vi "He magnet field fpga.vi"() -> ()   [LabVIEW 2016]
uses:
  <vilib>/LabVIEW Targets/FPGA/cRIO/shared/nicrio_ModuleControls/nicrio_cRIO-9871_BaudRateEnum.ctl
  <vilib>/LabVIEW Targets/FPGA/cRIO/shared/nicrio_ModuleControls/nicrio_cRIO-9871_DataBitsEnum.ctl
  <vilib>/LabVIEW Targets/FPGA/cRIO/shared/nicrio_ModuleControls/nicrio_cRIO-9871_ParityEnum.ctl
  <vilib>/LabVIEW Targets/FPGA/cRIO/shared/nicrio_ModuleControls/nicrio_cRIO-9871_StopBitsEnum.ctl
  <vilib>/Platform/TimedLoop/XDataNode/timing_clust.ctl
  <vilib>/Platform/TimedLoop/XDataNode/nitl_modes.ctl
  <vilib>/Platform/TimedLoop/XDataNode/wakeup.ctl
  <vilib>/rvi/FXPMathLib/basic elements/FxpIntAccumulator/subVIs/nifxpmath_IntAccumulator_SimConfig.ctl
  <vilib>/rvi/Emulation/niFpgaGetClockAttributes.vi
  <vilib>/rvi/Emulation/niFpgaSctlEmulationGetInTimedLoop.vi
  <vilib>/rvi/Emulation/niFpgaEmulationReportErrorSimple.vi
  <vilib>/rvi/eio/common/nirviEmuTemplateMethod_errors.vi
  <vilib>/rvi/Emulation/niFpgaCriticalErrorInLSC.vi
  <vilib>/rvi/Analysis/common/codeGenErrors/XNode/niFpgaXNodeCodeGenErrorHandle.vi
  <vilib>/rvi/FXPMathLib/basic elements/FxpIntAccumulator/simVIs/DllFxpIntAccumulator_sub.vi
  <vilib>/rvi/eio/common/nirviEmuTemplatePropertySet_noerrors.vi
  <vilib>/eio/EIONode/EIONode.xnode
  <vilib>/eio/EIOMethodNode/EIOMethodNode.xnode
  <vilib>/rvi/Analysis/measure/dc-rms/XNode/niFpgaDC-RMS.xnode
  <vilib>/Platform/TimedLoop/XDataNode/XDataNode.xnode
  <vilib>/rvi/FXPMathLib/basic elements/FxpIntAccumulator/XNode/nifxpmath_IntAccumulator.xnode
  <vilib>/rvi/FXPMathLib/FxpMul/XNode/nifxpmath_Multiplier.xnode
  <vilib>/eio/EIOPropertyNode/EIOPropertyNode.xnode
  <vilib>/Platform/TimedLoop/XDataNode/XDNodeRunTimeDep.lvlib
  <vilib>/rvi/FXPMathLib/sim/FxpSim.dll
  <vilib>/rvi/eio/common/nirviEmuTemplatePropertyGet_errors.vi
  <vilib>/rvi/eio/common/nirviEmuTemplatePropertyGet_noerrors.vi
  <vilib>/rvi/eio/common/nirviEmuTemplatePropertySet_errors.vi
panel:
  out "Ion gauge 4":u8[](array[numeric])
  out "Convectron 4":u8[](array[numeric])
  out "Convectron 3":u8[](array[numeric])
  out "Ion gauge 3":u8[](array[numeric])
  out "Ion gauge 2":u8[](array[numeric])
  out "Convectron 2":u8[](array[numeric])
  out "Convectron 1":u8[](array[numeric])
  out "Ion gauge 1":u8[](array[numeric])
  in  "Analyze Image FC":bool
  in  "Tank Exit FC":bool
  out "Analyze Out?":bool
  out "Analyze IN?":bool
  in  "Analog Output":fxp<+/-,26,5>[](array[numeric])=[0.0, 0.0, 0.0, 0.0, 0.0, 0.0, 0.0, 0.0] format="%.23g"
  out "Analog input":fxp<+/-,26,5>[](array[numeric]) format="%.23g"
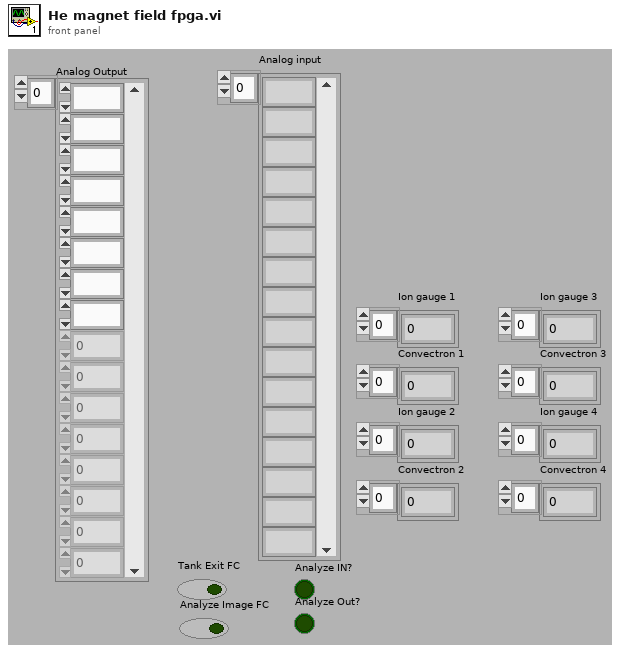
[diagram p1: front panel]
types:
  T1 = typedef "nicrio_cRIO-9871_StopBitsEnum.ctl" = enum8{"1", "1.5", "2"}
  T2 = typedef "nicrio_cRIO-9871_ParityEnum.ctl" = enum8{"None", "Odd", "Even", "Mark", "Space"}
  T3 = typedef "nicrio_cRIO-9871_DataBitsEnum.ctl" = enum8{"5", "6", "7", "8"}
  T4 = typedef "nicrio_cRIO-9871_BaudRateEnum.ctl" = enum16{"75 bps", "110 bps", "134 bps", "150 bps", "300 bps", "600 bps", "1200 bps", "1800 bps", "2400 bps", "4800 bps", "7200 bps", "9600 bps", "14.4 kbps", "19.2 kbps", "28.8 kbps", "38.4 kbps", "57.6 kbps", "115.2 kbps", "230.4 kbps", "460.8 kbps", "921.6 kbps"}
  T5 = typedef "XDNodeRunTimeDep.lvlib/timing_clust.ctl" = cluster{"Expected End [f-1]":u64, "Actual End [f-1]":u64, "Finished Late? [f-1]":bool, "Expected End [i-1]":u64, "Actual End [i-1]":u64, "Finished Late? [i-1]":bool, "Expected Start [i]":u64, "Actual Start [i]":u64, "Expected Start [f]":u64, "Actual Start [f]":u64, "Source Name":string, "Structure Name":string, "Period":i64, "Deadline":i64, "Offset":i64, "Start":i64, "Priority":i32, "Timeout":i32, "Mode":T6, "Wakeup Reason":T7, "Error":errorcluster, "Source Type":string, "Secondary Source Type":string, "Global End Time":u64, "Global Start Time":u64, "Frame Duration":u64, "Iteration Duration":u64, "Assigned CPU":i32, "I/O Scan Engine Mode":u32}
  T6 = typedef "XDNodeRunTimeDep.lvlib/nitl_modes.ctl" = enum32{"No Change", "Process missed periods, maintain original phase", "Discard missed periods, maintain original phase", "Process missed periods, ignore original phase", "Discard missed periods, ignore original phase"}
  T7 = typedef "XDNodeRunTimeDep.lvlib/wakeup.ctl" = enum32{"Normal", "Aborted", "Asynchronous wakeup", "Timing source error", "Timed loop error", "Timeout"}
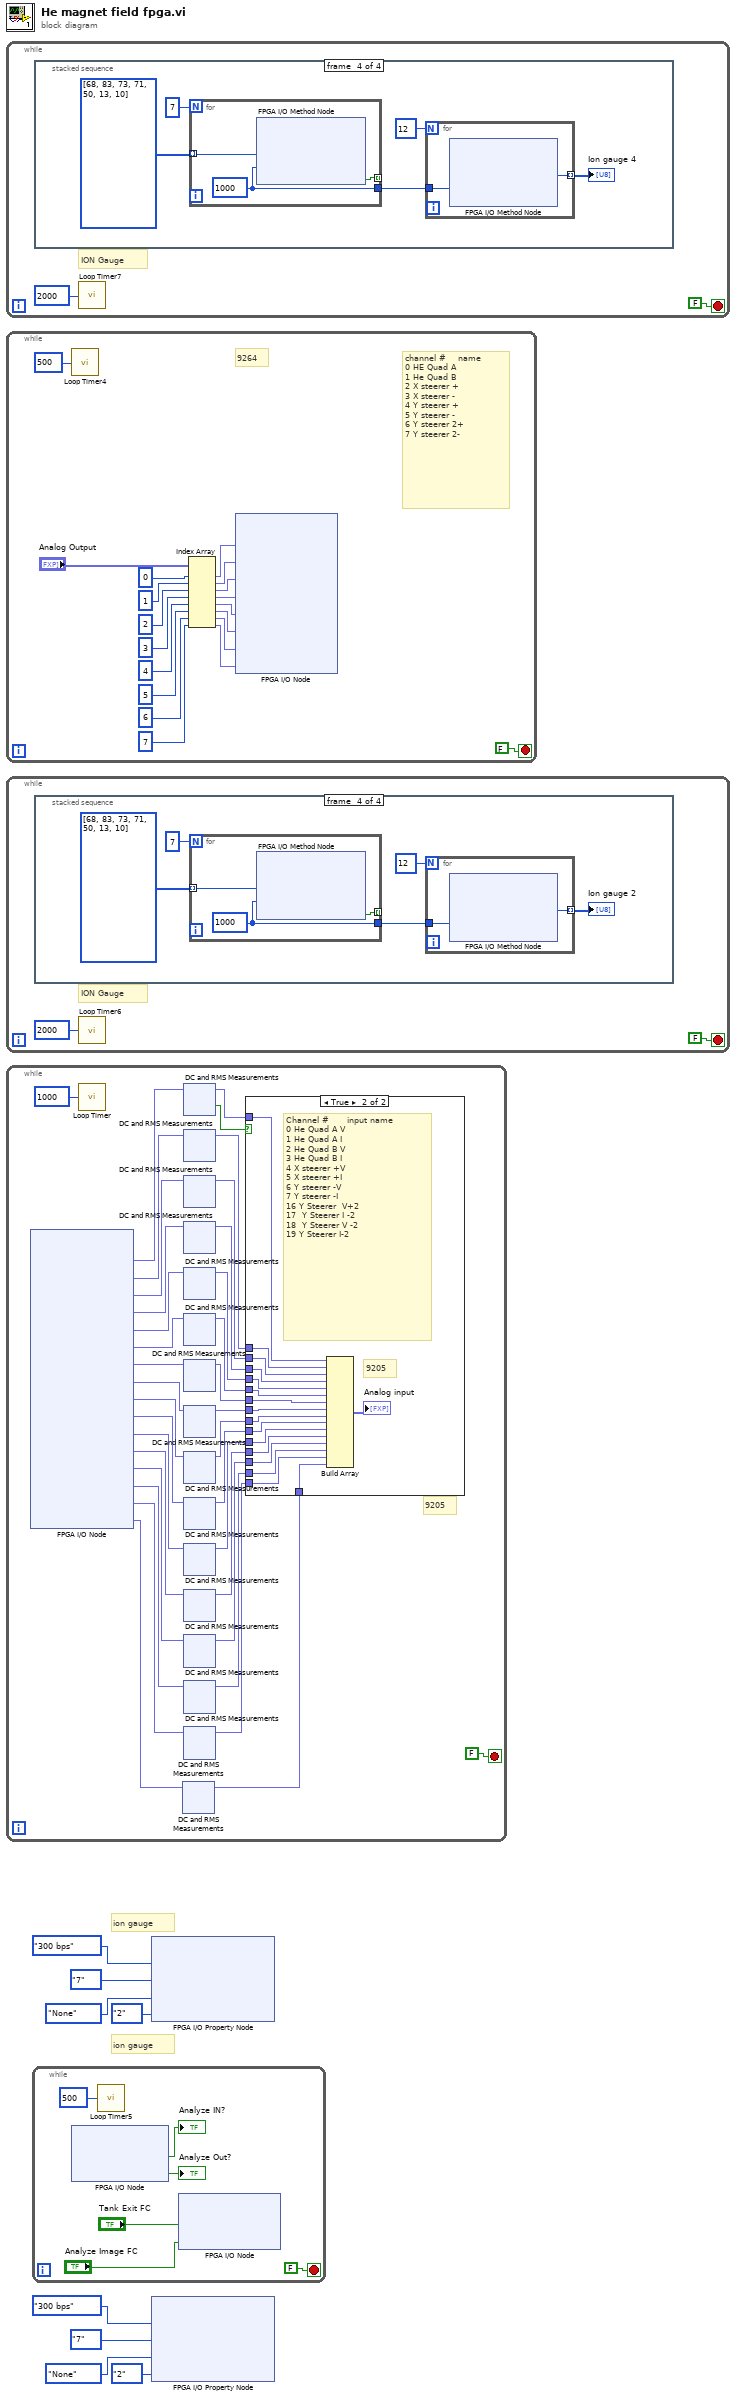
[diagram p0: block diagram]
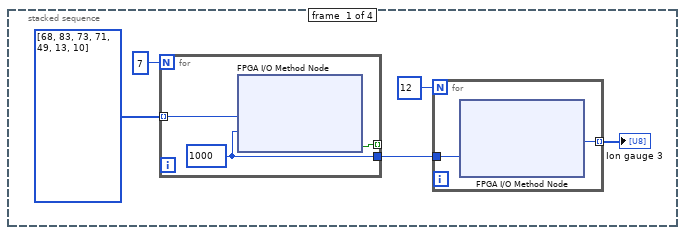
[diagram p3: hidden frame]
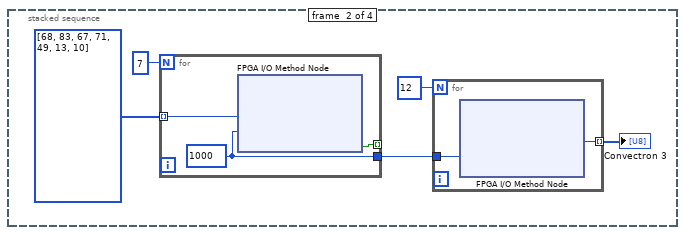
[diagram p4: hidden frame]
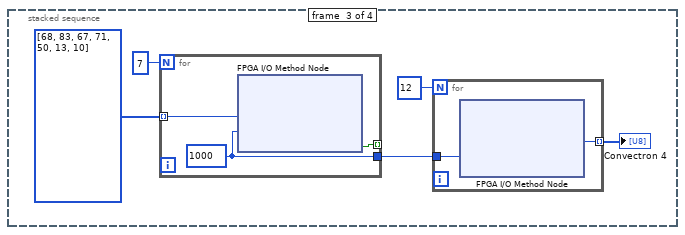
[diagram p5: hidden frame]
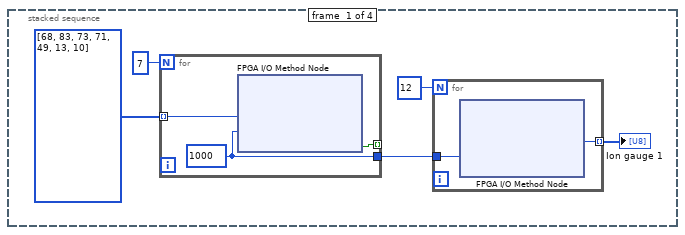
[diagram p6: hidden frame]
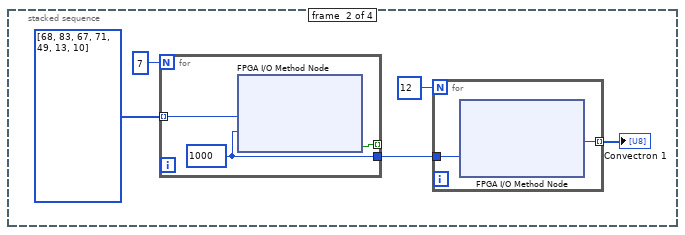
[diagram p7: hidden frame]
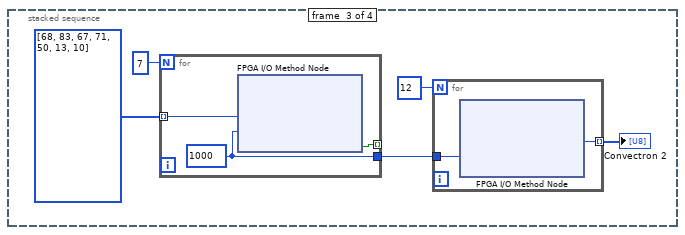
[diagram p8: hidden frame]
diagram:
  # "ion gauge"
  # "ion gauge"
  n1 = while {
    stop <- FALSE stop-if-true
    # "ION Gauge"
    n2 = stacked-sequence {
      frame #0 {
        n3 = for {
          N: 7 -> [_]
          tunnel: [w18] -> w15
          tunnel: [w19] -> _ mode=indexing
          tunnel: u8[] [68, 83, 73, 71, 49, 13, 10] ("unsigned byte array") -> [w20] mode=indexing
          w18 = 1000 ("Timeout (ms)")
          n4 = xnode "FPGA I/O Method Node"("Data"=w20, "Timeout (ms)"=w18) -> ("Timed Out"=w19:bool)  [unwired: 1 in, 1 out]
        }
        n5 = for {
          N: 12 -> [_]
          tunnel: w15 -> [w17]
          tunnel: [w16] -> w11 mode=indexing
          n6 = xnode "FPGA I/O Method Node"("Timeout (ms)"=w17) -> ("Data"=w16:u8)  [unwired: 1 in, 2 out]
        }
        "Ion gauge 3" <- w11
      }
      frame #1 {
        n7 = for {
          N: 7 -> [_]
          tunnel: [w29] -> w25
          tunnel: [w28] -> _ mode=indexing
          tunnel: u8[] [68, 83, 67, 71, 49, 13, 10] ("unsigned byte array") -> [w30] mode=indexing
          w29 = 1000 ("Timeout (ms)")
          n8 = xnode "FPGA I/O Method Node"("Data"=w30, "Timeout (ms)"=w29) -> ("Timed Out"=w28:bool)  [unwired: 1 in, 1 out]
        }
        n9 = for {
          N: 12 -> [_]
          tunnel: w25 -> [w26]
          tunnel: [w27] -> w21 mode=indexing
          n10 = xnode "FPGA I/O Method Node"("Timeout (ms)"=w26) -> ("Data"=w27:u8)  [unwired: 1 in, 2 out]
        }
        "Convectron 3" <- w21
      }
      frame #2 {
        n11 = for {
          N: 7 -> [_]
          tunnel: [w38] -> w35
          tunnel: [w39] -> _ mode=indexing
          tunnel: u8[] [68, 83, 67, 71, 50, 13, 10] ("unsigned byte array") -> [w40] mode=indexing
          w38 = 1000 ("Timeout (ms)")
          n12 = xnode "FPGA I/O Method Node"("Data"=w40, "Timeout (ms)"=w38) -> ("Timed Out"=w39:bool)  [unwired: 1 in, 1 out]
        }
        n13 = for {
          N: 12 -> [_]
          tunnel: w35 -> [w37]
          tunnel: [w36] -> w31 mode=indexing
          n14 = xnode "FPGA I/O Method Node"("Timeout (ms)"=w37) -> ("Data"=w36:u8)  [unwired: 1 in, 2 out]
        }
        "Convectron 4" <- w31
      }
      frame #3 {
        n15 = for {
          N: 7 -> [_]
          tunnel: [w49] -> w45
          tunnel: [w48] -> _ mode=indexing
          tunnel: u8[] [68, 83, 73, 71, 50, 13, 10] ("unsigned byte array") -> [w50] mode=indexing
          w49 = 1000 ("Timeout (ms)")
          n16 = xnode "FPGA I/O Method Node"("Data"=w50, "Timeout (ms)"=w49) -> ("Timed Out"=w48:bool)  [unwired: 1 in, 1 out]
        }
        n17 = for {
          N: 12 -> [_]
          tunnel: w45 -> [w47]
          tunnel: [w46] -> w41 mode=indexing
          n18 = xnode "FPGA I/O Method Node"("Timeout (ms)"=w47) -> ("Data"=w46:u8)  [unwired: 1 in, 2 out]
        }
        "Ion gauge 4" <- w41
      }
    }
    n19 = call "Loop Timer7"("Count(mSec)"=u32 2000 ("Count(Ticks)")) -> ()  [unwired: 1 out]
  }
  n20 = while {
    stop <- FALSE stop-if-true
    # "channel #    name\n0 HE Quad A\n1 He Quad B\n2 X steerer +\n3 X steerer -\n4 Y steerer +\n5 Y steerer -\n6 Y steerer 2+\n7 Y steerer 2-"
    # "9264"
    n21 = call "Loop Timer4"("Count(uSec)"=u32 500 ("Count(Ticks)")) -> ()  [unwired: 1 out]
    n22 = Index Array(array="Analog Output", index #1=0 ("index"), index #2=1 ("index"), index #3=2 ("index"), index #4=3 ("index"), index #5=4 ("index"), index #6=5 ("index"), index #7=6 ("index"), index #8=7 ("index")) -> (element #1=w62:fxp<+/-,26,5>, element #2=w61:fxp<+/-,26,5>, element #3=w60:fxp<+/-,26,5>, element #4=w59:fxp<+/-,26,5>, element #5=w54:fxp<+/-,26,5>, element #6=w53:fxp<+/-,26,5>, element #7=w52:fxp<+/-,26,5>, element #8=w51:fxp<+/-,26,5>)
    n23 = xnode "FPGA I/O Node"("Mod1/AO0"=w62, "Mod1/AO1"=w61, "Mod1/AO2"=w60, "Mod1/AO3"=w59, "Mod1/AO4"=w54, "Mod1/AO5"=w53, "Mod1/AO6"=w52, "Mod1/AO7"=w51) -> ()  [unwired: 8 in, 8 out]
  }
  n24 = while {
    stop <- FALSE stop-if-true
    # "ION Gauge"
    n25 = stacked-sequence {
      frame #0 {
        n26 = for {
          N: 7 -> [_]
          tunnel: [w80] -> w76
          tunnel: [w79] -> _ mode=indexing
          tunnel: u8[] [68, 83, 73, 71, 49, 13, 10] ("unsigned byte array") -> [w81] mode=indexing
          w80 = 1000 ("Timeout (ms)")
          n27 = xnode "FPGA I/O Method Node"("Data"=w81, "Timeout (ms)"=w80) -> ("Timed Out"=w79:bool)  [unwired: 1 in, 1 out]
        }
        n28 = for {
          N: 12 -> [_]
          tunnel: w76 -> [w78]
          tunnel: [w77] -> w72 mode=indexing
          n29 = xnode "FPGA I/O Method Node"("Timeout (ms)"=w78) -> ("Data"=w77:u8)  [unwired: 1 in, 2 out]
        }
        "Ion gauge 1" <- w72
      }
      frame #1 {
        n30 = for {
          N: 7 -> [_]
          tunnel: [w90] -> w86
          tunnel: [w89] -> _ mode=indexing
          tunnel: u8[] [68, 83, 67, 71, 49, 13, 10] ("unsigned byte array") -> [w91] mode=indexing
          w90 = 1000 ("Timeout (ms)")
          n31 = xnode "FPGA I/O Method Node"("Data"=w91, "Timeout (ms)"=w90) -> ("Timed Out"=w89:bool)  [unwired: 1 in, 1 out]
        }
        n32 = for {
          N: 12 -> [_]
          tunnel: w86 -> [w88]
          tunnel: [w87] -> w82 mode=indexing
          n33 = xnode "FPGA I/O Method Node"("Timeout (ms)"=w88) -> ("Data"=w87:u8)  [unwired: 1 in, 2 out]
        }
        "Convectron 1" <- w82
      }
      frame #2 {
        n34 = for {
          N: 7 -> [_]
          tunnel: [w100] -> w96
          tunnel: [w99] -> _ mode=indexing
          tunnel: u8[] [68, 83, 67, 71, 50, 13, 10] ("unsigned byte array") -> [w101] mode=indexing
          w100 = 1000 ("Timeout (ms)")
          n35 = xnode "FPGA I/O Method Node"("Data"=w101, "Timeout (ms)"=w100) -> ("Timed Out"=w99:bool)  [unwired: 1 in, 1 out]
        }
        n36 = for {
          N: 12 -> [_]
          tunnel: w96 -> [w98]
          tunnel: [w97] -> w92 mode=indexing
          n37 = xnode "FPGA I/O Method Node"("Timeout (ms)"=w98) -> ("Data"=w97:u8)  [unwired: 1 in, 2 out]
        }
        "Convectron 2" <- w92
      }
      frame #3 {
        n38 = for {
          N: 7 -> [_]
          tunnel: [w110] -> w106
          tunnel: [w109] -> _ mode=indexing
          tunnel: u8[] [68, 83, 73, 71, 50, 13, 10] ("unsigned byte array") -> [w111] mode=indexing
          w110 = 1000 ("Timeout (ms)")
          n39 = xnode "FPGA I/O Method Node"("Data"=w111, "Timeout (ms)"=w110) -> ("Timed Out"=w109:bool)  [unwired: 1 in, 1 out]
        }
        n40 = for {
          N: 12 -> [_]
          tunnel: w106 -> [w108]
          tunnel: [w107] -> w102 mode=indexing
          n41 = xnode "FPGA I/O Method Node"("Timeout (ms)"=w108) -> ("Data"=w107:u8)  [unwired: 1 in, 2 out]
        }
        "Ion gauge 2" <- w102
      }
    }
    n42 = call "Loop Timer6"("Count(mSec)"=u32 2000 ("Count(Ticks)")) -> ()  [unwired: 1 out]
  }
  n43 = while {
    stop <- FALSE stop-if-true
    # "9205"
    n44 = xnode "FPGA I/O Node"() -> ("Mod2/AI0"=w143:fxp<+/-,26,5>, "Mod2/AI1"=w141:fxp<+/-,26,5>, "Mod2/AI2"=w139:fxp<+/-,26,5>, "Mod2/AI3"=w137:fxp<+/-,26,5>, "Mod2/AI4"=w135:fxp<+/-,26,5>, "Mod2/AI5"=w133:fxp<+/-,26,5>, "Mod2/AI6"=w131:fxp<+/-,26,5>, "Mod2/AI7"=w129:fxp<+/-,26,5>, "Mod2/AI16"=w127:fxp<+/-,26,5>, "Mod2/AI17"=w125:fxp<+/-,26,5>, "Mod2/AI18"=w123:fxp<+/-,26,5>, "Mod2/AI19"=w121:fxp<+/-,26,5>, "Mod2/AI20"=w119:fxp<+/-,26,5>, "Mod2/AI21"=w117:fxp<+/-,26,5>, "Mod2/AI22"=w115:fxp<+/-,26,5>, "Mod2/AI23"=w113:fxp<+/-,26,5>)  [unwired: 16 in, 16 out]
    n45 = call "Loop Timer"("Count(Ticks)"=u32 1000) -> ()  [unwired: 1 out]
    n46 = xnode "DC and RMS Measurements"("input data"=w113) -> ("DC"=w112:fxp<+/-,26,5>)  [unwired: 1 in, 1 out]
    n47 = xnode "DC and RMS Measurements"("input data"=w143) -> ("DC"=w142:fxp<+/-,26,5>, "output valid"=w144:bool)  [unwired: 1 in]
    n48 = xnode "DC and RMS Measurements"("input data"=w141) -> ("DC"=w140:fxp<+/-,26,5>)  [unwired: 1 in, 1 out]
    n49 = xnode "DC and RMS Measurements"("input data"=w139) -> ("DC"=w138:fxp<+/-,26,5>)  [unwired: 1 in, 1 out]
    n50 = xnode "DC and RMS Measurements"("input data"=w137) -> ("DC"=w136:fxp<+/-,26,5>)  [unwired: 1 in, 1 out]
    n51 = xnode "DC and RMS Measurements"("input data"=w135) -> ("DC"=w134:fxp<+/-,26,5>)  [unwired: 1 in, 1 out]
    n52 = xnode "DC and RMS Measurements"("input data"=w133) -> ("DC"=w132:fxp<+/-,26,5>)  [unwired: 1 in, 1 out]
    n53 = xnode "DC and RMS Measurements"("input data"=w131) -> ("DC"=w130:fxp<+/-,26,5>)  [unwired: 1 in, 1 out]
    n54 = xnode "DC and RMS Measurements"("input data"=w129) -> ("DC"=w128:fxp<+/-,26,5>)  [unwired: 1 in, 1 out]
    n55 = xnode "DC and RMS Measurements"("input data"=w127) -> ("DC"=w126:fxp<+/-,26,5>)  [unwired: 1 in, 1 out]
    n56 = xnode "DC and RMS Measurements"("input data"=w125) -> ("DC"=w124:fxp<+/-,26,5>)  [unwired: 1 in, 1 out]
    n57 = xnode "DC and RMS Measurements"("input data"=w123) -> ("DC"=w122:fxp<+/-,26,5>)  [unwired: 1 in, 1 out]
    n58 = xnode "DC and RMS Measurements"("input data"=w121) -> ("DC"=w120:fxp<+/-,26,5>)  [unwired: 1 in, 1 out]
    n59 = xnode "DC and RMS Measurements"("input data"=w119) -> ("DC"=w118:fxp<+/-,26,5>)  [unwired: 1 in, 1 out]
    n60 = xnode "DC and RMS Measurements"("input data"=w117) -> ("DC"=w116:fxp<+/-,26,5>)  [unwired: 1 in, 1 out]
    n61 = xnode "DC and RMS Measurements"("input data"=w115) -> ("DC"=w114:fxp<+/-,26,5>)  [unwired: 1 in, 1 out]
    n62 = case shown="True" w144 {
      tunnel: w142 -> [_ w403]
      tunnel: w140 -> [_ w402]
      tunnel: w138 -> [_ w401]
      tunnel: w136 -> [_ w400]
      tunnel: w134 -> [_ w399]
      tunnel: w132 -> [_ w398]
      tunnel: w130 -> [_ w397]
      tunnel: w128 -> [_ w396]
      tunnel: w126 -> [_ w395]
      tunnel: w124 -> [_ w394]
      tunnel: w122 -> [_ w393]
      tunnel: w120 -> [_ w392]
      tunnel: w118 -> [_ w391]
      tunnel: w116 -> [_ w390]
      tunnel: w114 -> [_ w389]
      tunnel: w112 -> [_ w387]
      frame False {
      }
      frame True {
        # "Channel #      input name\n0 He Quad A V\n1 He Quad A I\n2 He Quad B V\n3 He Quad B I\n4 X steerer +V\n5 X steerer +I\n6 Y steerer -V\n7 Y steerer -I\n16 Y Steerer  V+2\n17  Y Steerer I -2\n18  Y Steerer V -2\n19 Y Steerer I-2"
        # "9205"
        n63 = Build Array(w403, w402, w401, w400, w399, w398, w397, w396, w395, w394, w393, w392, w391, w390, w389, w387) -> (→"Analog input":fxp<+/-,26,5>[])
      }
    }
  }
  n64 = while {
    stop <- FALSE stop-if-true
    n65 = xnode "FPGA I/O Node"() -> ("Mod7/DI0"=→"Analyze IN?":bool, "Mod7/DI1"=→"Analyze Out?":bool)  [unwired: 2 in, 2 out]
    n66 = call "Loop Timer5"("Count(mSec)"=u32 500 ("Count(Ticks)")) -> ()  [unwired: 1 out]
    n67 = xnode "FPGA I/O Node"("Mod8/CH0"="Tank Exit FC", "Mod8/CH1"="Analyze Image FC") -> ()  [unwired: 2 in, 2 out]
  }
  n68 = xnode "FPGA I/O Property Node"("Baud Rate"=nicrio_cRIO-9871_BaudRateEnum."300 bps", "Data Bits"=nicrio_cRIO-9871_DataBitsEnum."7", "Parity"=nicrio_cRIO-9871_ParityEnum."None", "Stop Bits"=nicrio_cRIO-9871_StopBitsEnum."2") -> ()  [unwired: 1 in, 1 out]
  n69 = xnode "FPGA I/O Property Node"("Baud Rate"=nicrio_cRIO-9871_BaudRateEnum."300 bps", "Data Bits"=nicrio_cRIO-9871_DataBitsEnum."7", "Parity"=nicrio_cRIO-9871_ParityEnum."None", "Stop Bits"=nicrio_cRIO-9871_StopBitsEnum."2") -> ()  [unwired: 1 in, 1 out]
